vi "Write queue to stdin.vi"(8 "error in (no error)":errorcluster, 10 "queue in":refnum<queue>, 11 "subprocess in":refnum<class "Buffered Subprocess.lvclass">) -> (0 "error out":errorcluster, 2 "queue out":refnum<queue>, 3 "subprocess out":refnum<class "Buffered Subprocess.lvclass">)   [LabVIEW 2020, in "NI_Subprocess.lvlib" / "Buffered Subprocess.lvclass"]
uses:
  <vilib>/Subprocess/Buffered Subprocess/Buffered Subprocess.lvclass
  <vilib>/Array/Bytestream/Bytestream.lvclass
  <vilib>/Subprocess/Buffered Subprocess/Buffered Subprocess.lvclass/Buffered Subprocess.ctl
  49b2f372-b0ea-3fed-7fb1-21231282e53f.vi
  <vilib>/Array/Bytestream/Concatenate Array.vi
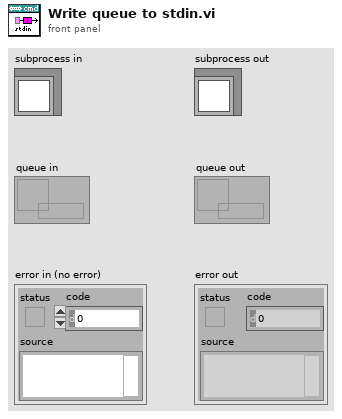
[diagram p1: front panel]
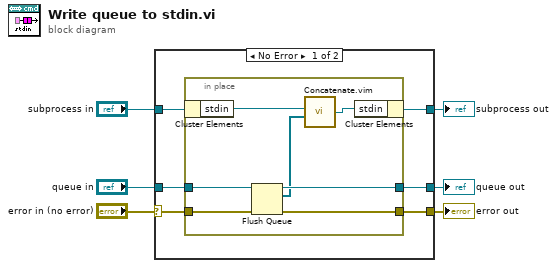
[diagram p0: block diagram]
diagram:
  n1 = case shown="No Error" "error in (no error)" {
    selector: "error in (no error)" -> [w10 w22]
    tunnel: [w7 w22] -> w5
    tunnel: [w8 w21] -> w3
    tunnel: "subprocess in" -> [w12 w21]
    tunnel: "queue in" -> [w11 w20]
    tunnel: [w9 w20] -> w1
    frame No Error {
      n2 = in-place {
        in-place-border: w11 -> [w19]
        in-place-border: w10 -> [w18]
        in-place-border: [w17] -> w9
        in-place-border: [w13] -> w7
        n3 = in-place-cluster #1(w12) -> ("stdin"=w16:refnum<class "Bytestream.lvclass">)
        n4 = Flush Queue(queue=w19, error in (no error)=w18) -> (queue out=w17:refnum<queue>, remaining elements=w15:refnum<class "Bytestream.lvclass">[], error out=w13:errorcluster)
        n5 = call "Concatenate.vim"("b"=w15, "a"=w16) -> ("a+b"=w14:refnum<class "Bytestream.lvclass">)  [unwired: 2 in]
        n6 = in-place-cluster #1("stdin"=w14) -> (w8:refnum<class "Buffered Subprocess.lvclass">)
      }
    }
    frame Error {
    }
  }
  "error out" <- w5
  "subprocess out" <- w3
  "queue out" <- w1
